vi "Initialize Attributes.vi"(8 "error in (no error)":errorcluster, 10 "Attribute Data":variant, 11 "CS++OPCUAInterface in":refnum<class "CS++OPCUAInterface.lvclass">) -> (0 "error out":errorcluster, 2 "Found?":bool, 3 "CS++OPCUAInterface out":refnum<class "CS++OPCUAInterface.lvclass">)   [LabVIEW 2015, in "CS++OPCUAInterface.lvlib" / "CS++OPCUAInterface.lvclass"]
doc: "Initialize object attribute.\n\nUnique resources should be allocated elsewhere!"
uses:
  CS++OPCUAInterface.lvclass
  CSPP_Core/Actors/CS++BaseActor/CS++BaseActor.lvclass/CS++BaseActor.ctl
  CS++OPCUAInterface.lvclass/CS++OPCUAInterface.ctl
  CSPP_Core/Actors/CS++BaseActor/Read CS++Factory.vi
  CSPP_Core/Actors/CS++BaseActor/Read Object Name.vi
  CSPP_Core/Actors/CS++BaseActor/CS++BaseActor.lvclass
  CSPP_Core/Classes/CS++BaseClasses/Factory/CS++Factory.lvclass
  <vilib>/OPCUA/NI OPC UA Utility.lvlib
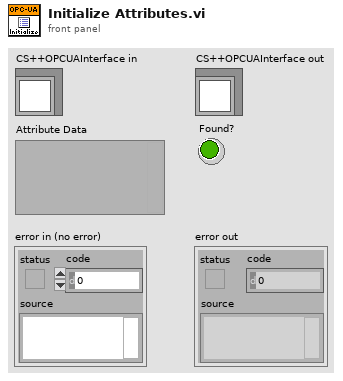
[diagram p1: front panel]
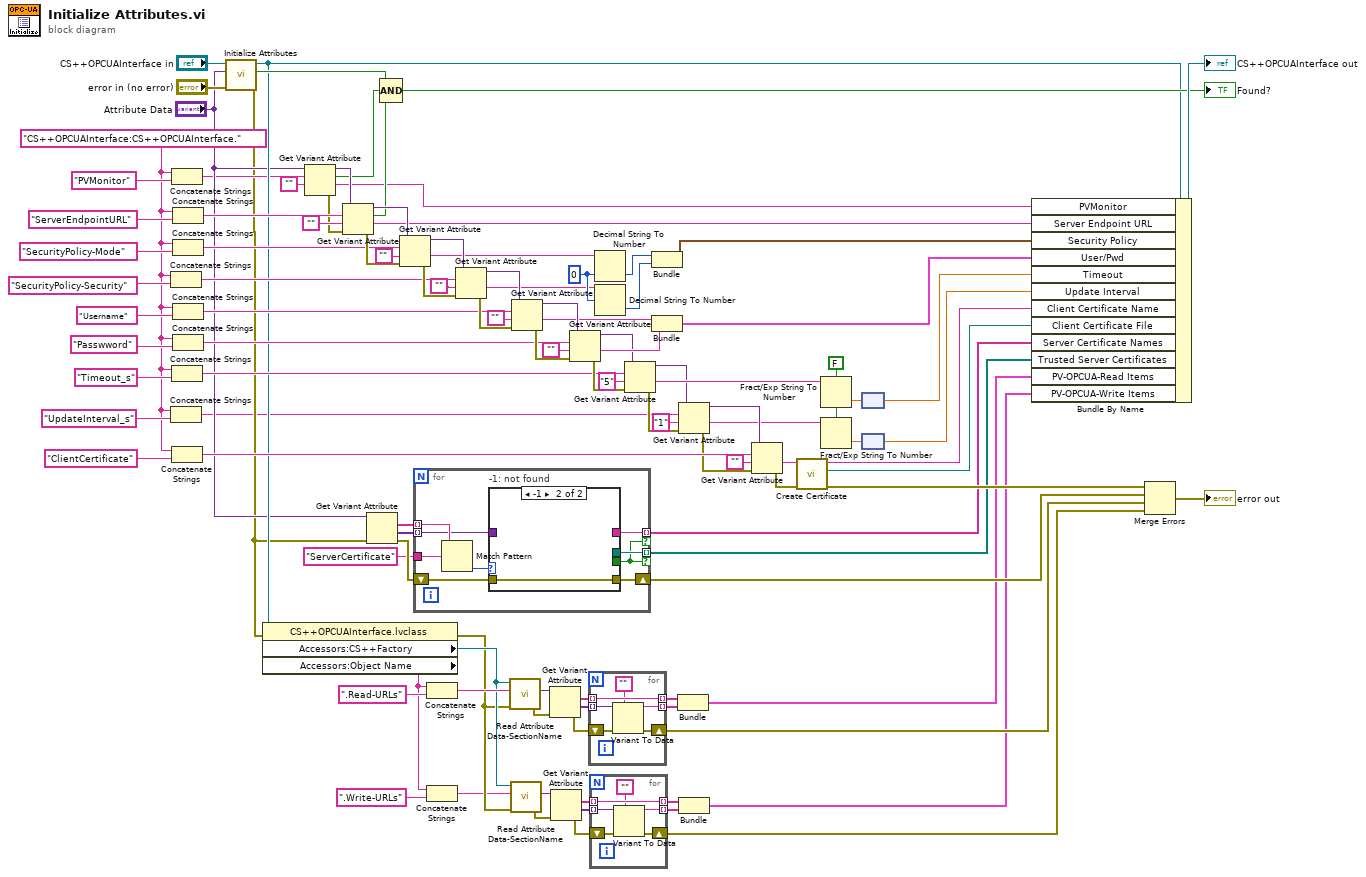
[diagram p0: block diagram]
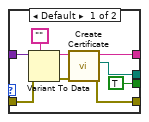
[diagram p2: hidden frame]
diagram:
  w25 = u16 0
  w3 = FALSE ("use system decimal point (T)")
  w5 = "CS++OPCUAInterface:CS++OPCUAInterface." ("string")
  n1 = Concatenate Strings(w5, "SecurityPolicy-Security" ("string")) -> (w96:string)
  n2 = Concatenate Strings(w5, "UpdateInterval_s" ("string")) -> (w6:string)
  n3 = Concatenate Strings(w5, "PVMonitor" ("string")) -> (w17:string)
  n4 = Concatenate Strings(w5, "Timeout_s" ("string")) -> (w75:string)
  n5 = Concatenate Strings(w5, "ClientCertificate" ("string")) -> (w70:string)
  n6 = Concatenate Strings(w5, "ServerEndpointURL" ("string")) -> (w107:string)
  n7 = Concatenate Strings(w5, "SecurityPolicy-Mode" ("string")) -> (w99:string)
  n8 = Concatenate Strings(w5, "Username" ("string")) -> (w93:string)
  n9 = Concatenate Strings(w5, "Passwword" ("string")) -> (w82:string)
  n10 = call-parent "Initialize Attributes.vi"("error in (no error)"="error in (no error)", "Attribute Data"="Attribute Data", "CS++BaseActor in"="CS++OPCUAInterface in") -> ("error out"=w16:errorcluster, "Found?"=w57:bool, "CS++BaseActor out"=w54:refnum<class "CS++OPCUAInterface.lvclass">)  [unwired: 6 in]
  n11 = property class="CS++OPCUAInterface.lvclass"(reference=w54, error in=w16) -> (error out=w32:errorcluster, "Accessors:CS++Factory"=w33:refnum<class "CS++Factory.lvclass">, "Accessors:Object Name"=w52:string)  [unwired: 1 out]
  n12 = Get Variant Attribute(Variant="Attribute Data", name=w17, default value (empty Variant)="") -> (duplicate Variant=w20:variant, found=w13:bool, value=w14:string, error out=w15:errorcluster)  [unwired: 1 in]
  n13 = Get Variant Attribute(Variant=w20, name=w107, default value (empty Variant)="", error in=w15) -> (duplicate Variant=w105:variant, found=w90:bool, value=w91:string, error out=w104:errorcluster)
  n14 = Get Variant Attribute(Variant="Attribute Data", error in=w16) -> (names=w65:string[], values=w64:variant[], error out=w63:errorcluster)  [unwired: 2 in, 1 out]
  n15 = Compound Arithmetic op=AND(w57, w13, w90) -> (→"Found?":bool)
  n16 = Get Variant Attribute(Variant=w105, name=w99, default value (empty Variant)="", error in=w104) -> (duplicate Variant=w98:variant, value=w27:string, error out=w97:errorcluster)  [unwired: 1 out]
  n17 = for {
    tunnel: w65 -> [w119] mode=indexing
    tunnel: w64 -> [w117] mode=indexing
    shift-right: [w114] -> w60
    shift-left: w63 -> [w116]
    tunnel: "ServerCertificate" ("string") -> [w118]
    tunnel: [w113] -> w59 mode=indexing if=w111
    tunnel: [w112] -> w58 mode=indexing if=w111
    n18 = Match Pattern(string=w119, regular expression=w118) -> (offset past match=w115:i32)  [unwired: 1 in, 3 out]
    n19 = case "-1: not found" shown="-1" w115 {
      tunnel: w117 -> [w128 _]
      tunnel: w116 -> [w126 w129]
      tunnel: [w122 w129] -> w114
      tunnel: [w123 _] -> w113
      tunnel: [w121 _] -> w112
      tunnel: [TRUE _] -> w111
      frame Default {
        n20 = Variant To Data(error in=w126, type="", Variant=w128) -> (data=w124:string, error out=w125:errorcluster)
        n21 = call <vilib>:"Create Certificate.vi"("error in (no error)"=w125, "certificate name in"=w124) -> ("error out"=w122:errorcluster, "certificate path"=w121:path, "certificate name out"=w123:string)  [unwired: 6 in, 1 out]
      }
      frame -1 {
      }
    }
  }
  n22 = Concatenate Strings(w52, ".Read-URLs" ("string")) -> (w44:string)
  n23 = Concatenate Strings(w52, ".Write-URLs" ("string")) -> (w31:string)
  n24 = Get Variant Attribute(Variant=w98, name=w96, default value (empty Variant)="", error in=w97) -> (duplicate Variant=w95:variant, value=w23:string, error out=w94:errorcluster)  [unwired: 1 out]
  n25 = call-dynamic "Read Attribute Data-SectionName.vi"("error in (no error)"=w32, "Object Name"=w44, "CS++Factory in"=w33) -> ("error out"=w47:errorcluster, "Attribute Data"=w49:variant)  [unwired: 6 in, 1 out]
  n26 = call-dynamic "Read Attribute Data-SectionName.vi"("error in (no error)"=w32, "Object Name"=w31, "CS++Factory in"=w33) -> ("error out"=w36:errorcluster, "Attribute Data"=w34:variant)  [unwired: 6 in, 1 out]
  n27 = Get Variant Attribute(Variant=w95, name=w93, default value (empty Variant)="", error in=w94) -> (duplicate Variant=w84:variant, value=w81:string, error out=w83:errorcluster)  [unwired: 1 out]
  n28 = Get Variant Attribute(Variant=w49, error in=w47) -> (names=w45:string[], values=w48:variant[], error out=w46:errorcluster)  [unwired: 2 in, 1 out]
  n29 = Get Variant Attribute(Variant=w34, error in=w36) -> (names=w38:string[], values=w35:variant[], error out=w37:errorcluster)  [unwired: 2 in, 1 out]
  n30 = Get Variant Attribute(Variant=w84, name=w82, default value (empty Variant)="", error in=w83) -> (duplicate Variant=w77:variant, value=w80:string, error out=w76:errorcluster)  [unwired: 1 out]
  n31 = for {
    tunnel: w48 -> [w133] mode=indexing
    tunnel: w45 -> [w134] mode=indexing
    tunnel: [w134] -> w43 mode=indexing
    tunnel: [w131] -> w42 mode=indexing
    shift-right: [w130] -> w50
    shift-left: w46 -> [w135]
    n32 = Variant To Data(error in=w135, type="", Variant=w133) -> (data=w131:string, error out=w130:errorcluster)
  }
  n33 = for {
    tunnel: w35 -> [w139] mode=indexing
    tunnel: w38 -> [w140] mode=indexing
    tunnel: [w140] -> w39 mode=indexing
    tunnel: [w137] -> w40 mode=indexing
    shift-right: [w136] -> w29
    shift-left: w37 -> [w141]
    n34 = Variant To Data(error in=w141, type="", Variant=w139) -> (data=w137:string, error out=w136:errorcluster)
  }
  n35 = Decimal String To Number(string=w27, default (0L)=w25) -> (number=w26:u16)  [unwired: 1 in, 1 out]
  n36 = Decimal String To Number(string=w23, offset=w25) -> (number=w22:i32)  [unwired: 1 in, 1 out]
  n37 = Get Variant Attribute(Variant=w77, name=w75, default value (empty Variant)="5", error in=w76) -> (duplicate Variant=w7:variant, value=w74:string, error out=w11:errorcluster)  [unwired: 1 out]
  n38 = Bundle(w26, w22) -> (w89:cluster{u16, i32})  [unwired: 1 in]
  n39 = Bundle(w81, w80) -> (w79:cluster{string, string})  [unwired: 1 in]
  n40 = Bundle(w43, w42) -> (w41:cluster{string[], string[]})  [unwired: 1 in]
  n41 = Get Variant Attribute(Variant=w7, name=w6, default value (empty Variant)="1" ("name"), error in=w11) -> (duplicate Variant=w12:variant, value=w2:string, error out=w10:errorcluster)  [unwired: 1 out]
  n42 = Bundle(w39, w40) -> (w30:cluster{string[], string[]})  [unwired: 1 in]
  n43 = Get Variant Attribute(Variant=w12, name=w70, default value (empty Variant)="", error in=w10) -> (value=w69:string, error out=w68:errorcluster)  [unwired: 2 out]
  n44 = call <vilib>:"Create Certificate.vi"("error in (no error)"=w68, "certificate name in"=w69) -> ("error out"=w61:errorcluster, "certificate path"=w67:path, "certificate name out"=w66:string)  [unwired: 6 in, 1 out]
  n45 = Fract/Exp String To Number(use system decimal point (T)=w3, string=w74) -> (number=w73:dbl)  [unwired: 2 in, 1 out]
  n46 = Fract/Exp String To Number(use system decimal point (T)=w3, string=w2) -> (number=w4:dbl)  [unwired: 2 in, 1 out]
  n47 = node(w73) -> (w72:dbl[unit])
  n48 = node(w4) -> (w1:dbl[unit])
  n49 = Bundle By Name(cluster=w54, "PVMonitor"=w14, "Server Endpoint URL"=w91, "Security Policy"=w89, "User/Pwd"=w79, "Timeout"=w72, "Update Interval"=w1, "Client Certificate Name"=w66, "Client Certificate File"=w67, "Server Certificate Names"=w59, "Trusted Server Certificates"=w58, "PV-OPCUA-Read Items"=w41, "PV-OPCUA-Write Items"=w30) -> (→"CS++OPCUAInterface out":refnum<class "CS++OPCUAInterface.lvclass">)
  n50 = Merge Errors(w61, w60, w50, w29) -> (→"error out":errorcluster)
